vi "FABR-Plot Thresholds.vi"(0 "Analysis":T1, 2 "Neural Ref":refnum<vi>, 11 "error in (no error)":errorcluster) -> (15 "error out":errorcluster)   [LabVIEW 2020]
uses:
  Typedefs/FABR-Analysis State.ctl
  epl-vi-lib/Utility VIs/Math VIs/LinSpace (x0-dx-npts).vi
  epl-vi-lib/Utility VIs/Math VIs/interp1.vi
panel:
  # "Freq X Level X Time"
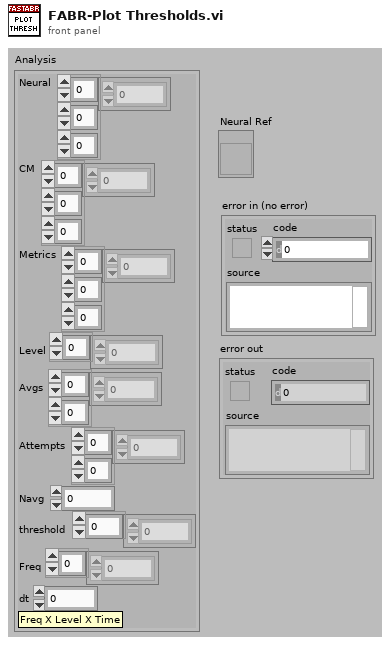
[diagram p1: front panel]
types:
  T1 = typedef "FABR-Analysis State.ctl" = cluster{"Neural":dbl[][][], "CM":dbl[][][], "Metrics":dbl[][][], "Level":dbl[], "Avgs":i32[][], "Attempts":i32[][], "Navg":i32, "threshold":dbl[], "Freq":dbl[], "dt":dbl}
  T2 = typedef "LVRectTypeDef.ctl" = cluster{"Left":i16, "Top":i16, "Right":i16, "Bottom":i16}
  T3 = cluster{"Width":i16, "Style":enum32{"Solid", "Dash", "Dot", "DashDot", "DashDotDot"}}
  T4 = typedef "LVPoint32TypeDef.ctl" = cluster{"Horizontal":i32, "Vertical":i32}
  T5 = cluster{"Horizontal":i32, i32, "Horizontal":i32, i32}
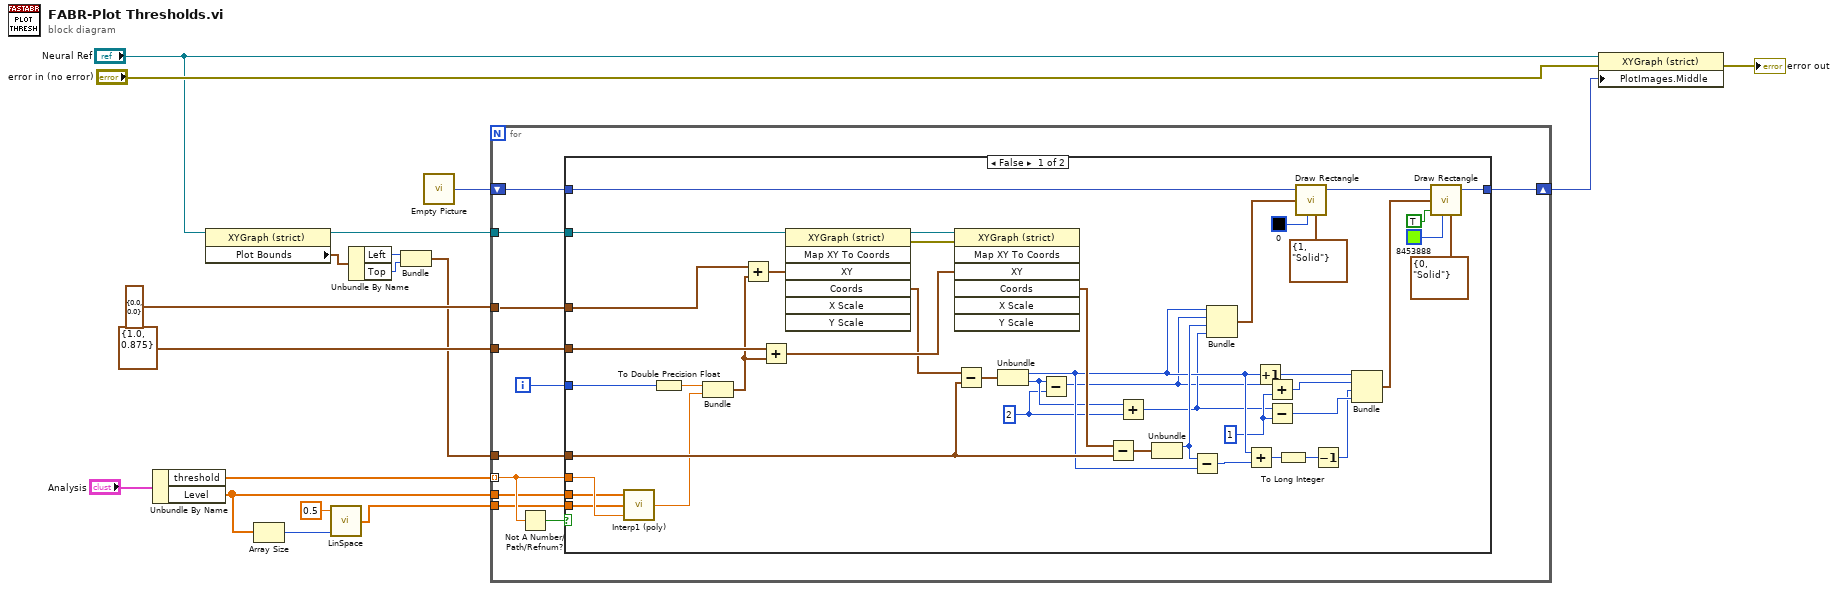
[diagram p0: block diagram]
diagram:
  n1 = Unbundle By Name("Analysis") -> ("threshold"=w15:dbl[], "Level"=w1:dbl[])
  n2 = property class="XYGraph (strict)"(reference="Neural Ref") -> (reference out=w10:refnum<vi>, "Plot Bounds"=w8:T2)  [unwired: 1 in, 1 out]
  n3 = Array Size(array=w1) -> (size(s)=w4:i32)
  n4 = call-poly "LinSpace.vi"("npts"=w4, "x0"=0.5) -> ("Array"=w2:dbl[])  [unwired: 2 in, 1 out]
  n5 = Unbundle By Name(w8) -> ("Left"=w7:i16, "Top"=w6:i16)
  n6 = Bundle("Left"=w7, "Top"=w6) -> (w5:cluster{"Left":i16, "Top":i16})  [unwired: 1 in]
  n7 = call "Empty Picture"() -> ("empty picture"=w14:picture)
  n8 = for {
    tunnel: w15 -> [w21] mode=indexing
    shift-right: [w28] -> w13
    shift-left: w14 -> [w29]
    tunnel: cluster{"X":dbl, "Y":dbl} {"X"=0.0, "Y"=0.0} ("XY") -> [w27]
    tunnel: w10 -> [w25]
    tunnel: cluster{"X":dbl, "Y":dbl} {"X"=1.0, "Y"=0.875} ("XY") -> [w24]
    tunnel: w5 -> [w23]
    tunnel: w2 -> [w20]
    tunnel: w1 -> [w19]
    i -> [w26]
    n9 = Not A Number/Path/Refnum?(number/path/refnum=w21) -> (NaN/Path/Refnum?=w22:bool)
    n10 = case shown="False" w22 {
      tunnel: w29 -> [w72 w73]
      tunnel: w27 -> [w71 _]
      tunnel: w26 -> [w70 _]
      tunnel: w25 -> [w68 _]
      tunnel: w24 -> [w65 _]
      tunnel: w23 -> [w58 _]
      tunnel: [w56 w73] -> w28
      tunnel: w21 -> [w39 _]
      tunnel: w20 -> [w38 _]
      tunnel: w19 -> [w37 _]
      frame False {
        w33 = 2 ("y")
        w43 = 1
        n11 = call-poly "Interp1 (poly).vi"("X"=w37, "Y"=w38, "U"=w39) -> ("V"=w36:dbl)  [unwired: 2 in]
        n12 = To Double Precision Float(number=w70) -> (double precision float=w35:dbl)
        n13 = Bundle(w35, "V"=w36) -> (w64:cluster{dbl, "V":dbl})  [unwired: 1 in]
        n14 = Add(x=w71, y=w64) -> (x+y=w69:cluster{dbl, dbl})
        n15 = Add(x=w65, y=w64) -> (x+y=w63:cluster{dbl, dbl})
        n16 = invoke class="XYGraph (strict)" method="Map XY To Coords"(reference=w68, "XY"=w69) -> (reference out=w67:refnum<vi>, error out=w66:errorcluster, "Coords"=w62:T4)  [unwired: 5 in, 4 out]
        n17 = invoke class="XYGraph (strict)" method="Map XY To Coords"(reference=w67, error in=w66, "XY"=w63) -> ("Coords"=w61:T4)  [unwired: 4 in, 6 out]
        n18 = Subtract(x=w62, y=w58) -> (x-y=w60:T4)
        n19 = Unbundle(w60) -> ("Horizontal"=w45:i32, "Vertical"=w34:i32)
        n20 = Subtract(x=w34, y=w33) -> (x-y=w41:i32)
        n21 = Subtract(x=w61, y=w58) -> (x-y=w59:T4)
        n22 = Add(x=w34, y=w33) -> (x+y=w42:i32)
        n23 = Unbundle(w59) -> ("Horizontal"=w53:i32)  [unwired: 1 out]
        n24 = Subtract(x=w53, y=w45) -> (x-y=w51:i32)
        n25 = Bundle("Horizontal"=w45, w41, "Horizontal"=w53, w42) -> (w52:T5)  [unwired: 1 in]
        n26 = Add(x=w45, y=w51) -> (x+y=w49:i32)
        n27 = Increment(x=w45) -> (x+1=w31:i32)
        n28 = Add(x=w41, y=w43) -> (x+y=w50:i32)
        n29 = Subtract(x=w42, y=w43) -> (x-y=w47:i32)
        n30 = To Long Integer(number=w49) -> (32bit integer=w48:i32)
        n31 = call <vilib>:"Draw Rectangle.vi"("picture"=w72, "rect"=w52, "color(black)"=u32 0, "pen"=T3 {"Width"=1, "Style"=enum."Solid"}) -> ("new picture"=w57:picture)  [unwired: 5 in]
        n32 = Decrement(x=w48) -> (x-1=w30:i32)
        n33 = Bundle(w31, w50, w30, w47) -> (w46:cluster{i32, i32, i32, i32})  [unwired: 1 in]
        n34 = call <vilib>:"Draw Rectangle.vi"("picture"=w57, "rect"=w46, "fill?(F)"=TRUE, "color(black)"=u32 8453888, "pen"=T3 {"Width"=0, "Style"=enum."Solid"}) -> ("new picture"=w56:picture)  [unwired: 4 in]
      }
      frame True {
      }
    }
  }
  n35 = property class="XYGraph (strict)"(reference="Neural Ref", error in="error in (no error)", "PlotImages.Middle"=w13) -> (error out=→"error out":errorcluster)  [unwired: 1 out]
